vi "Pneu_Control.vi"(4 "Shooter_Arm":T1=enum."In", 5 "Flipper_Arb":enum16{"Closed", "Open"}(ring), 6 "Gear":bool, 7 "Intake Arm":T3=enum."Intake Portcullis") -> (0 "Gear Co mmand":T2, 1 "Flipper":T2, 2 "Shooter_Arm":T2, 3 "Intake_Arm":T2)   [LabVIEW 2015]
uses:
  Intake Enum..ctl
  <vilib>/Rock Robotics/WPI/Solenoid/WPI_SolenoidValue.ctl
  Arm_defense_Type_Def.ctl
  Global_Var/Drive_Global.vi
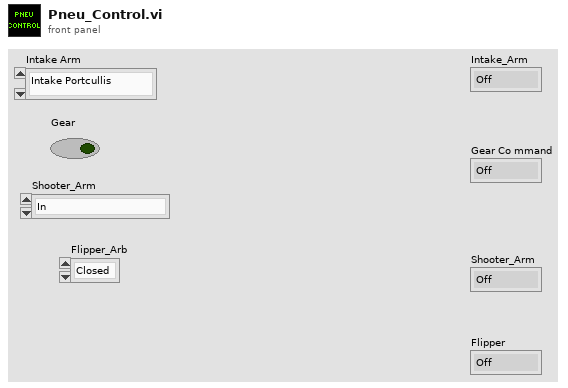
[diagram p1: front panel]
types:
  T1 = typedef "Arm_defense_Type_Def.ctl" = enum16{"Cheval de Frise", "Portcullis", "Out", "In", "Ball_Pickup"}
  T2 = typedef "WPI_SolenoidValue.ctl" = enum16{"Off", "On", "Forward", "Reverse"}
  T3 = typedef "Intake Enum..ctl" = enum16{"Float", "Intake Portcullis", "Intake Ball Pickup", "Intake Cheval", " Intake Raised"}
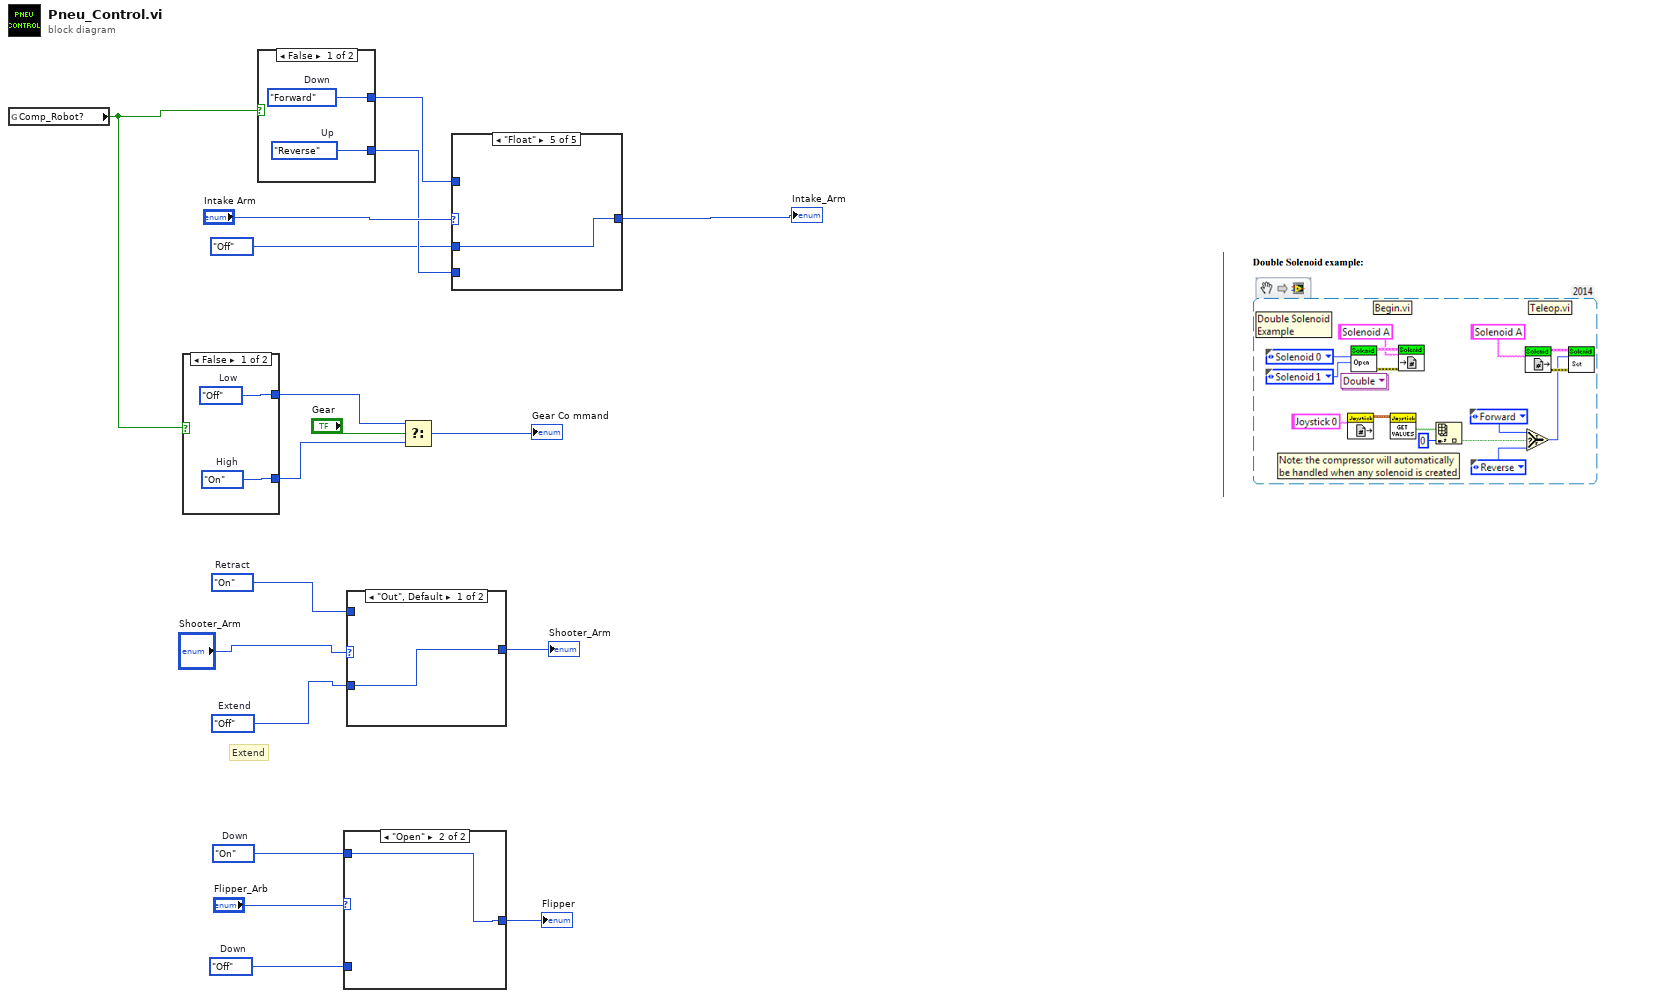
[diagram p0: block diagram]
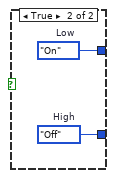
[diagram p3: hidden frame]
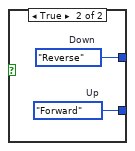
[diagram p4: hidden frame]
diagram:
  w10 = WPI_SolenoidValue."Off"  # Down
  w11 = WPI_SolenoidValue."On"  # Down
  w1 = WPI_SolenoidValue."Off"  # Extend
  w2 = WPI_SolenoidValue."On"  # Retract
  # "Extend"
  n1 = global read "Drive_Global.vi" "Comp_Robot?"() -> (w5:bool)
  n2 = case shown="False" w5 {
    tunnel: [w20 w22] -> w15
    tunnel: [w19 w21] -> w13
    frame False {
      w19 = WPI_SolenoidValue."On"  # High
      w20 = WPI_SolenoidValue."Off"  # Low
    }
    frame True {
      w21 = WPI_SolenoidValue."Off"  # High
      w22 = WPI_SolenoidValue."On"  # Low
    }
  }
  n3 = case shown="False" w5 {
    tunnel: [w24 w26] -> w17
    tunnel: [w23 w25] -> w16
    frame False {
      w23 = WPI_SolenoidValue."Reverse"  # Up
      w24 = WPI_SolenoidValue."Forward"  # Down
    }
    frame True {
      w25 = WPI_SolenoidValue."Forward"  # Up
      w26 = WPI_SolenoidValue."Reverse"  # Down
    }
  }
  n4 = case shown="\"Open\"" "Flipper_Arb" {
    tunnel: w11 -> [_ w28]
    tunnel: w10 -> [w27 _]
    tunnel: [w27 w28] -> w7
    frame "Closed", Default {
    }
    frame "Open" {
    }
  }
  "Flipper" <- w7
  n5 = case shown="\"Out\", Default" "Shooter_Arm" {
    tunnel: [w29 w30] -> w3
    tunnel: w2 -> [_ w30]
    tunnel: w1 -> [w29 _]
    frame "Out", Default {
    }
    frame "In" {
    }
  }
  "Shooter_Arm" <- w3
  n6 = Select(t=w15, s="Gear", f=w13) -> (s? t:f=→"Gear Co mmand":T2)
  n7 = case shown="\"Float\"" "Intake Arm" {
    tunnel: w17 -> [w31 w32 w33 _ _]
    tunnel: w16 -> [_ _ _ w34 _]
    tunnel: [w31 w32 w33 w34 w35] -> w6
    tunnel: WPI_SolenoidValue."Off" -> [_ _ _ _ w35]
    frame "Intake Portcullis", Default {
    }
    frame "Intake Ball Pickup" {
    }
    frame "Intake Cheval" {
    }
    frame " Intake Raised" {
    }
    frame "Float" {
    }
  }
  "Intake_Arm" <- w6
